vi "Get Hood LUT.vi"() -> (2 "Info":cluster{i32, i32}, 3 "LUT Out":i32[](array[numeric]))   [LabVIEW 2025]
panel:
  in  "Hood LUT":i32[](array[numeric])=[3, 5, 7, 9, 11]
  in  "Outputs":cluster{"Min Setpoint":i32, "Max Setpoint":i32}
  out "Max Hood Setpoint":i32
  out "Min Hood Setpoint":i32
  # "(number of teeth up from gear)"
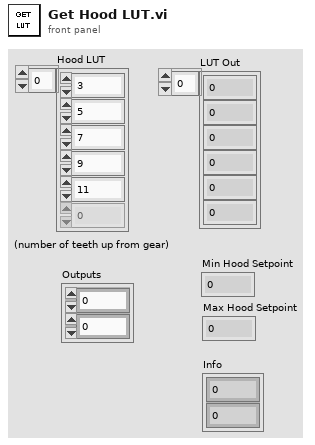
[diagram p1: front panel]
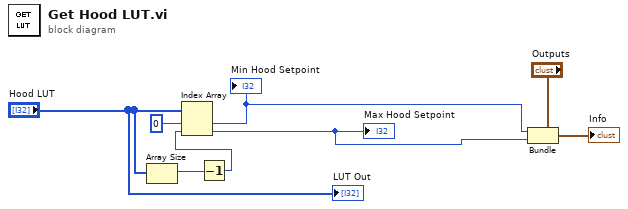
[diagram p0: block diagram]
diagram:
  n1 = Array Size(array="Hood LUT") -> (size(s)=w7:i32)
  n2 = Decrement(x=w7) -> (x-1=w5:i32)
  n3 = Index Array(array="Hood LUT", index #1=0 ("index"), index #2=w5) -> (element #1=w6:i32, element #2=w4:i32)
  "Min Hood Setpoint" <- w6
  "Max Hood Setpoint" <- w4
  n4 = Bundle(cluster="Outputs", "Min Setpoint"=w6, "Max Setpoint"=w4) -> (→"Info":cluster{"Min Setpoint":i32, "Max Setpoint":i32})
  "LUT Out" <- "Hood LUT"
